vi "测试-灰度变换Math Lookup.vi"() -> ()   [LabVIEW 2018]
doc: "This example shows how to apply a lookup table to an image. Lookup table (LUT) transformations are basic mathematical functions that can be used to improve the contrast and brightness of an image by modifying the intensity dynamics of regions with poor contrast. The LUT can also be used to highlight details in areas containing significant information. In NI Vision, apart from the predefined functions that can be used through the IMAQ MathLookup VI, you can also apply your own lookup tables using the IMAQ UserLookup VI."
uses:
  <vilib>/vision/NI_Vision_Development_Module.lvlib
  Dll/Otsu.dll
panel:
  out "Hist-label":T1(graph)
  out "labeled":T2(plugin-control) caption="Lut Image"
  out "# of Particles found":i32
  in  "Connectivity":bool
  out "Region Reports":T3(array[cluster]) {"Mean Value" format="%.2f"; "%" format="%.2f"; "Area (calibrated)" format="%.2f"; "Maximal Value" format="%.2f"; "Minimal Value" format="%.2f"; "Standard Variation" format="%.2f"}
  in  "Threshold Values":T4(slide)={"Minimum Value"=0.0, "Maximum Value"=65.106384} scale=0.0..255.0
  in  "Stop":bool
  out "Otsu":T2(plugin-control) caption="Lut Image"
  in  "灰度变化的区间设置":cluster{"Minimum":sgl, "Maximum":sgl}={"Minimum"=150.0, "Maximum"=255.0}
  out "Hist-Dst":T1(graph)
  out "H-Src":T1(graph)
  in  "完成灰度变换":bool
  in  "灰度变换模式选择":u16(ring)=3 items=["Log", "Linear", "Exp", "Square", "Square root", "Power X", "Power 1/X"]
  in  "X for Power X, 1/X":sgl=1.5 min=0 format="%_3g"
  out "LUT Image":T2(plugin-control) caption="Lut Image"
  out "Image Source":T2(plugin-control)
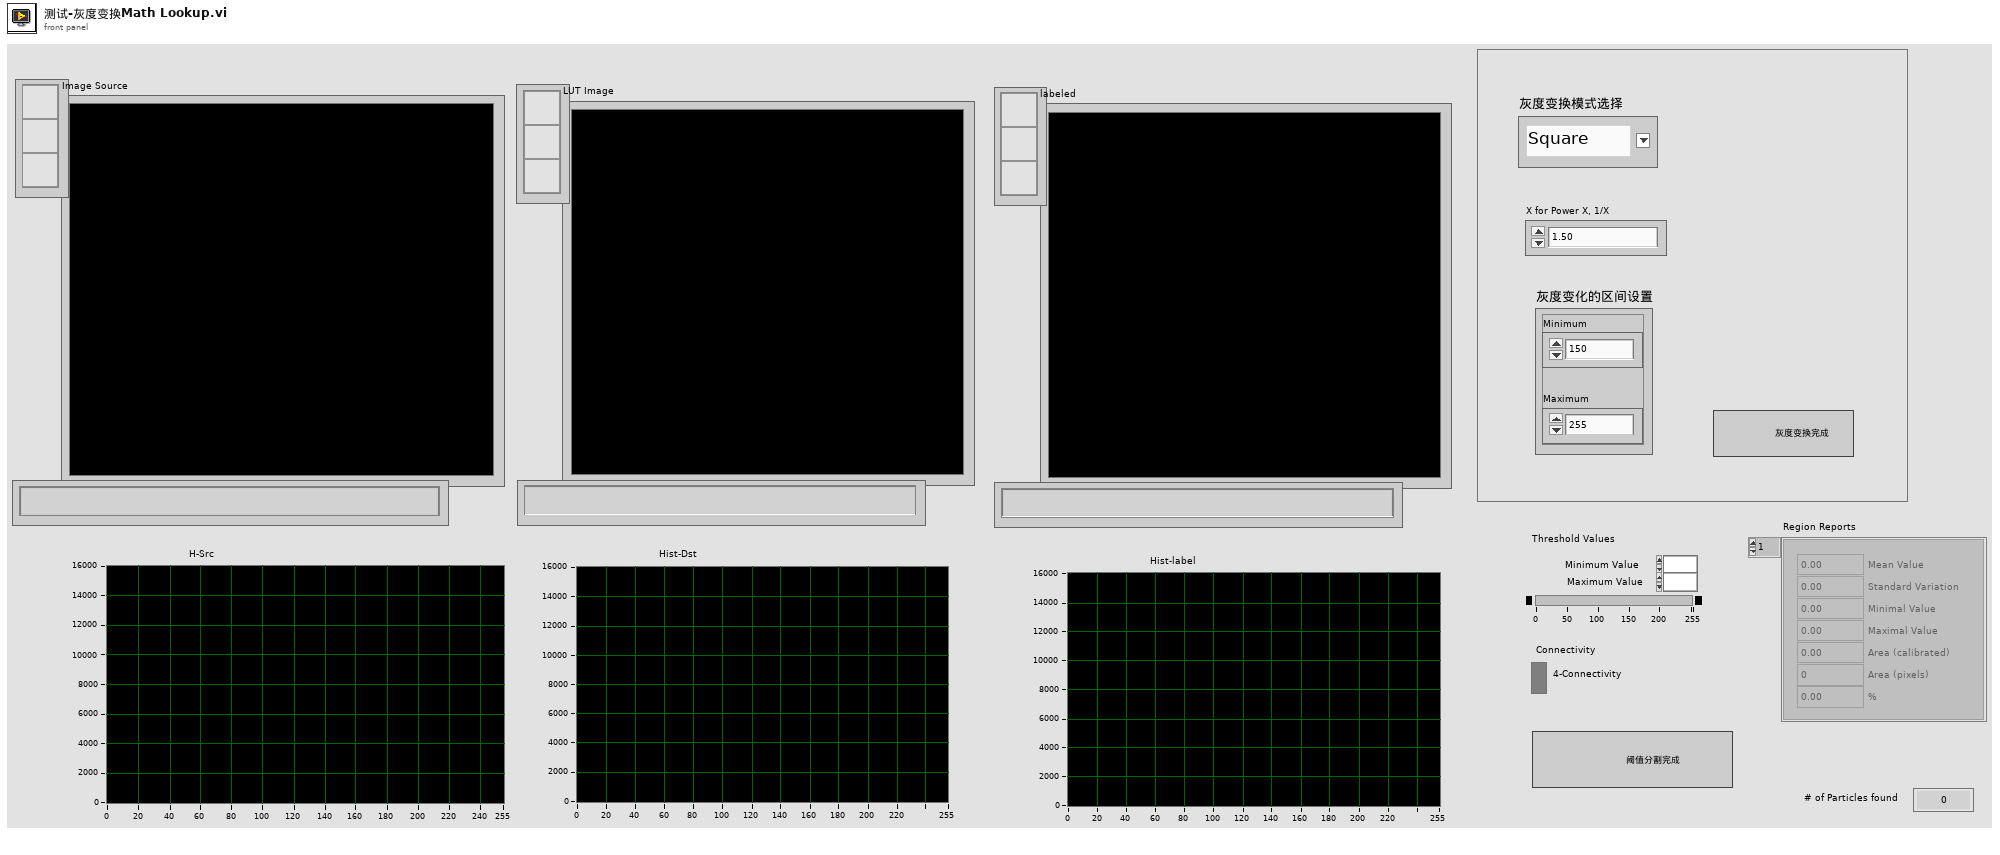
[diagram p1: front panel]
types:
  T1 = cluster{"Starting Value":sgl, "Incremental Value":sgl, "Histogram":u32[]}
  T2 = typedef "IMAQ Image.ctl" = refnum<image>
  T3 = cluster{"Mean Value":sgl, "Standard Variation":sgl, "Minimal Value":sgl, "Maximal Value":sgl, "Area (calibrated)":sgl, "Area (pixels)":i32, "%":sgl}[]
  T4 = cluster{"Minimum Value":sgl, "Maximum Value":sgl}
  T5 = typedef "Image Type" = u32
  T6 = enum32{"AutoM", "Close", "Dilate", "Erode", "Gradient", "Gradient out", "Gradient in", "Hit miss", "Open", "PClose", "POpen", "Thick", "Thin"}
  T7 = cluster{"X for Power X, 1/X":sgl, "灰度变换模式选择":u16}
  T8 = typedef "ROI Descriptor" = cluster{"Global Rectangle":i32[], "Contours":cluster{"ID":enum32{"External", "Internal"}, "Type":u32, "Coordinates":i32[]}[]}
  T9 = cluster{"Minimum Value":bool, "Maximum Value":bool}
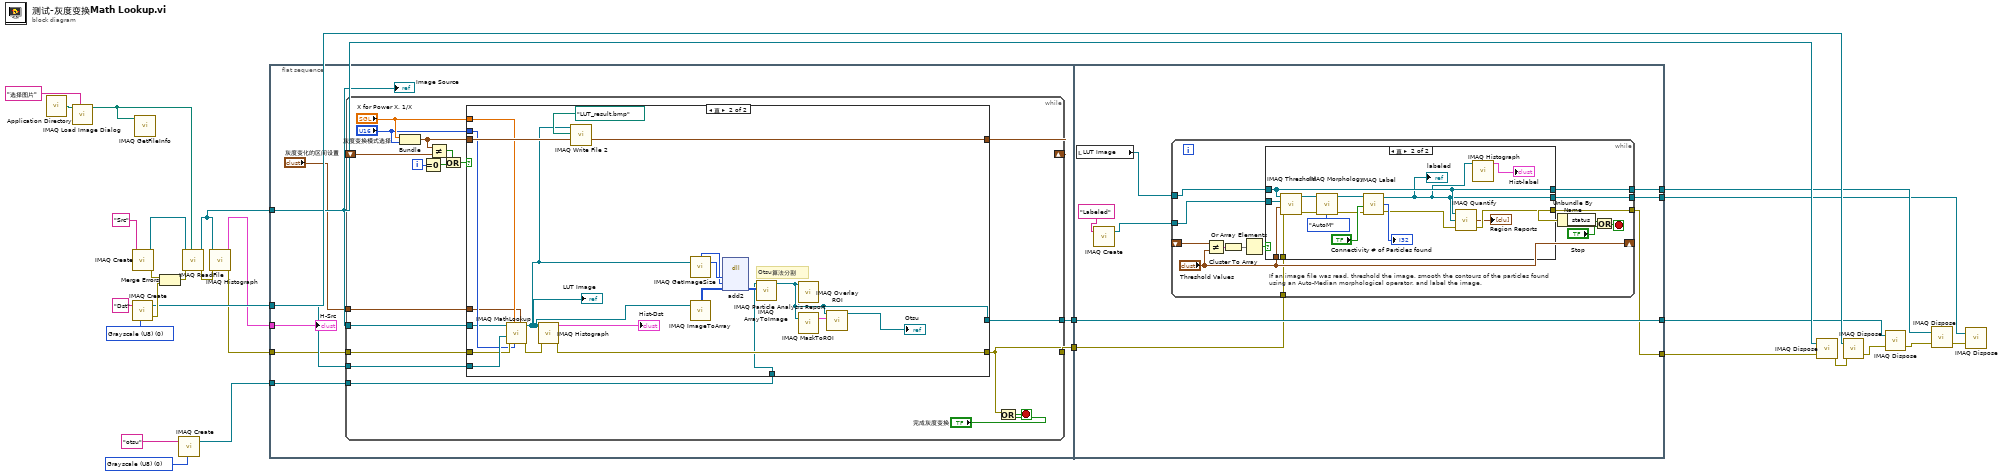
[diagram p0: block diagram]
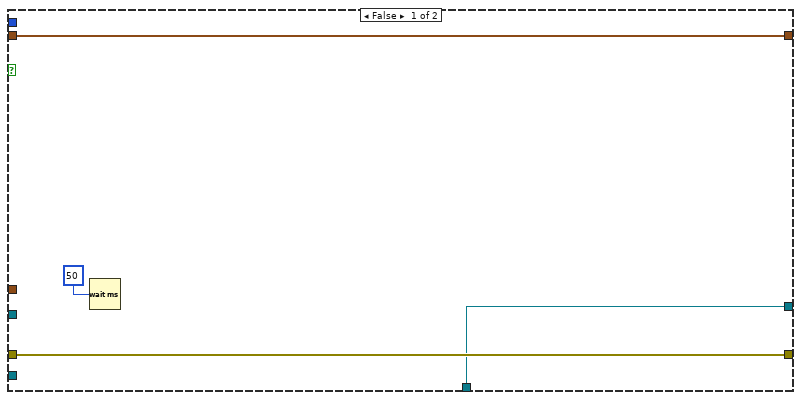
[diagram p2: hidden frame]
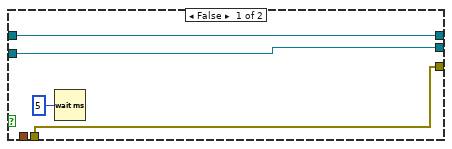
[diagram p3: hidden frame]
diagram:
  w11 = T5 0 items=["Grayscale (U8)", "Grayscale (I16)", "Grayscale (SGL)", "Complex (CSG)", "RGB (U32)", "HSL (U32)", "RGB (U64)", "Grayscale (U16)"] ("Image Type")
  w25 = T5 0 items=["Grayscale (U8)", "Grayscale (I16)", "Grayscale (SGL)", "Complex (CSG)", "RGB (U32)", "HSL (U32)", "RGB (U64)", "Grayscale (U16)"] ("Image Type")
  n1 = call <vilib>:"Application Directory.vi"() -> ("Application Directory"=w15:path)
  n2 = call "IMAQ Load Image Dialog"("Prompt"="选择图片" ("prompt"), "Start Path"=w15) -> ("Path"=w13:path)  [unwired: 7 in, 2 out]
  n3 = call "IMAQ Create"("Image Name"="Dst", "Image Type"=w25) -> ("New Image"=w21:T2, "error out"=w24:errorcluster)  [unwired: 3 in]
  n4 = call "IMAQ Create"("Image Name"="Src") -> ("New Image"=w27:T2, "error out"=w22:errorcluster)  [unwired: 4 in]
  n5 = call "IMAQ GetFileInfo"("File Path"=w13) -> ()  [unwired: 4 in, 7 out]
  n6 = Merge Errors(w22, w24) -> (w23:errorcluster)
  n7 = call "IMAQ Create"("Image Name"="otsu", "Image Type"=w11) -> ("New Image"=w10:T2)  [unwired: 3 in, 1 out]
  n8 = call "IMAQ ReadFile"("File Path"=w13, "error in (no error)"=w23, "Image"=w27) -> ("error out"=w19:errorcluster, "Image Out"=w18:T2)  [unwired: 4 in, 3 out]
  n9 = call "IMAQ Histograph"("error in (no error)"=w19, "Image"=w18) -> ("error out"=w17:errorcluster, "Histogram Graph"=w16:T1)  [unwired: 6 in, 2 out]
  n10 = flat-sequence {
    tunnel: w21 -> [w36]
    tunnel: w18 -> [w35]
    tunnel: w17 -> [w34]
    tunnel: w16 -> [w33]
    tunnel: w10 -> [w31]
    tunnel: [w30] -> w6
    tunnel: [w29] -> w5
    tunnel: [w86] -> w4
    tunnel: w6 -> [w86]
    tunnel: w5 -> [w79]
    tunnel: [w82] -> w3
    tunnel: [w81] -> w2
    tunnel: [w80] -> w1
    frame #0 {
      n11 = while {
        tunnel: w34 -> [w54]
        tunnel: w35 -> [w37]
        tunnel: w36 -> [w53]
        shift-right: [w52] -> _
        shift-left: _ -> [w51]
        tunnel: [w45] -> w29
        tunnel: "灰度变化的区间设置" -> [w40]
        tunnel: w31 -> [w39]
        tunnel: [w38] -> w30
        i -> [w50]
        stop <- w44 stop-if-true
        n12 = Bundle("X for Power X, 1/X"="X for Power X, 1/X", "灰度变换模式选择"="灰度变换模式选择") -> (w41:T7)  [unwired: 1 in]
        n13 = Equal To 0?(x=w50) -> (x = 0?=w48:bool)
        n14 = Not Equal?(x=w41, y=w51) -> (x != y?=w49:bool)
        n15 = Or(x=w49, y=w48) -> (x .or. y?=w47:bool)
        n16 = case shown="真" w47 {
          tunnel: w54 -> [w58 w76]
          tunnel: w37 -> [_ w59]
          tunnel: w41 -> [w57 w78]
          tunnel: w53 -> [_ w77]
          tunnel: [w57 w78] -> w52
          tunnel: [w58 w72] -> w45
          tunnel: "X for Power X, 1/X" -> [_ w75]
          tunnel: "灰度变换模式选择" -> [_ w74]
          tunnel: w40 -> [_ w70]
          tunnel: w39 -> [w55 w64]
          tunnel: [w55 w61] -> w38
          frame False {
            n17 = Wait (ms)(milliseconds to wait=u32 50) -> ()  [unwired: 1 out]
          }
          frame True {
            # "Otsu算法分割"
            n18 = call "IMAQ MathLookup"("Range"=w70, "Operator"=w74, "X Value"=w75, "error in (no error)"=w76, "Image Dst"=w77, "Image Src"=w59) -> ("error out"=w73:errorcluster, "Image Dst Out"=w60:T2)  [unwired: 4 in]
            "LUT Image" <- w60
            n19 = call "IMAQ Histograph"("error in (no error)"=w73, "Image"=w60) -> ("error out"=w72:errorcluster, "Histogram Graph"=→"Hist-Dst":T1)  [unwired: 6 in, 2 out]
            n20 = call-poly "IMAQ Write File 2"("File Path"=path "LUT_result.bmp", "Image"=w60) -> ()  [unwired: 8 in, 2 out]
            n21 = call "IMAQ GetImageSize"("Image"=w60) -> ("Y Resolution"=w68:i32, "X Resolution"=w67:i32)  [unwired: 3 in, 1 out]
            n22 = call "IMAQ ImageToArray"("Image"=w60) -> ("Image Pixels (U8)"=w66:u8[][])  [unwired: 3 in, 4 out]
            n23 = dll-call lib="PTH2Aabs EMyGithub\tMyLabVIEW晨光项目代码DllOtsu.dll" fn="add2"("rows"=w68, "cols"=w67, "data"=w66) -> ("data"=w65:u8[][])  [unwired: 6 in, 2 out]
            n24 = call "IMAQ ArrayToImage"("Image Pixels (U8)"=w65, "Image"=w64) -> ("Image Out"=w61:T2)  [unwired: 8 in, 1 out]
            n25 = call "IMAQ Particle Analysis Report"("Image"=w61) -> ()  [unwired: 5 in, 6 out]
            n26 = call "IMAQ MaskToROI"("Image"=w61) -> ("ROI Descriptor"=w63:T8)  [unwired: 6 in, 2 out]
            n27 = call "IMAQ Overlay ROI"("ROI Descriptor"=w63, "Image"=w61) -> ("Image Out"=→"Otsu":T2)  [unwired: 8 in, 1 out]
          }
        }
        n28 = Or(x=w45, y="完成灰度变换") -> (x .or. y?=w44:bool)
      }
      "Image Source" <- w35
      "H-Src" <- w33
    }
    frame #1 {
      n29 = local read "LUT Image"() -> (w85:T2)
      n30 = call "IMAQ Create"("Image Name"="Labeled") -> ("New Image"=w84:T2)  [unwired: 4 in, 1 out]
      n31 = while {
        tunnel: w85 -> [w100]
        tunnel: w84 -> [w99]
        shift-right: ["Threshold Values"] -> _
        shift-left: _ -> [w98]
        tunnel: [w88] -> w82
        tunnel: [w89] -> w81
        tunnel: [w90] -> w80
        tunnel: w79 -> [w87]
        stop <- w92 stop-if-true
        # "If an image file was read, threshold the image, smooth the contours of the particles found using an Auto-Median morphological operator, and label the image."
        n32 = Not Equal?(x=w98, y="Threshold Values") -> (x != y?=w97:T9)
        n33 = Cluster To Array(cluster=w97) -> (array=w96:bool[])
        n34 = Or Array Elements(Boolean array=w96) -> (logical OR=w95:bool)
        n35 = case shown="真" w95 {
          tunnel: w100 -> [w102 w109]
          tunnel: w99 -> [w103 w115]
          tunnel: "Threshold Values" -> [_ w112]
          tunnel: [w101 w110] -> w90
          tunnel: [w103 w107] -> w89
          tunnel: [w102 w109] -> w88
          tunnel: w87 -> [w101 w105]
          frame False {
            n36 = Wait (ms)(milliseconds to wait=u32 5) -> ()  [unwired: 1 out]
          }
          frame True {
            n37 = call "IMAQ Threshold"("error in (no error)"=w105, "Range"=w112, "Image Dst"=w115, "Image Src"=w109) -> ("error out"=w114:errorcluster, "Image Dst Out"=w119:T2)  [unwired: 6 in]
            n38 = call "IMAQ Morphology"("error in (no error)"=w114, "Operation"=T6."AutoM", "Image Src"=w119) -> ("error out"=w113:errorcluster, "Image Dst Out"=w116:T2)  [unwired: 7 in]
            n39 = call "IMAQ Label"("error in (no error)"=w113, "Connectivity 4/8 (8)"="Connectivity", "Image Src"=w116) -> ("error out"=w111:errorcluster, "Number of Particles"=→"# of Particles found":i32, "Image Dst Out"=w107:T2)  [unwired: 1 in]
            "labeled" <- w107
            n40 = call "IMAQ Quantify"("error in (no error)"=w111, "Image Mask"=w107, "Image"=w109) -> ("error out"=w110:errorcluster, "Region Reports"=→"Region Reports":T3)  [unwired: 1 out]
            n41 = call "IMAQ Histograph"("Image"=w107) -> ("Histogram Graph"=→"Hist-label":T1)  [unwired: 7 in, 3 out]
          }
        }
        n42 = Unbundle By Name(w90) -> ("status"=w94:bool)
        n43 = Or(x=w94, y="Stop") -> (x .or. y?=w92:bool)
      }
    }
  }
  n44 = call "IMAQ Dispose"("Image"=w18, "error in (no error)"=w1) -> ("error out"=w20:errorcluster)  [unwired: 4 in]
  n45 = call "IMAQ Dispose"("Image"=w21, "error in (no error)"=w20) -> ("error out"=w9:errorcluster)  [unwired: 4 in]
  n46 = call "IMAQ Dispose"("Image"=w4, "error in (no error)"=w9) -> ("error out"=w8:errorcluster)  [unwired: 4 in]
  n47 = call "IMAQ Dispose"("Image"=w3, "error in (no error)"=w8) -> ("error out"=w7:errorcluster)  [unwired: 4 in]
  n48 = call "IMAQ Dispose"("Image"=w2, "error in (no error)"=w7) -> ()  [unwired: 4 in, 1 out]
